vi "autoselect.vi"() -> (1 "60 Goal?":bool, 2 "Offense?":bool)   [LabVIEW 2012, in "Serenity_mk2.lvrbt"]
uses:
  Serenity_mk2.lvrbt
  <vilib>/NXT/Block Support/NXT_ButtonSelector.ctl
  <vilib>/NXT/Dual Mode Library/Display/drawText.vi
  <vilib>/NXT/Dual Mode Library/Sensors/readNXTButton.vi
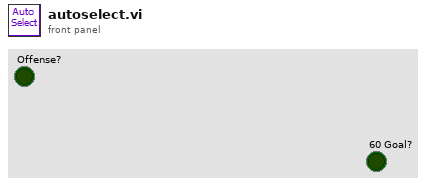
[diagram p1: front panel]
types:
  T1 = typedef "NXT_ButtonSelector.ctl" = u16
  T2 = typedef "LVHSConnector.ctl" = refnum<class "BrickReference.lvclass">
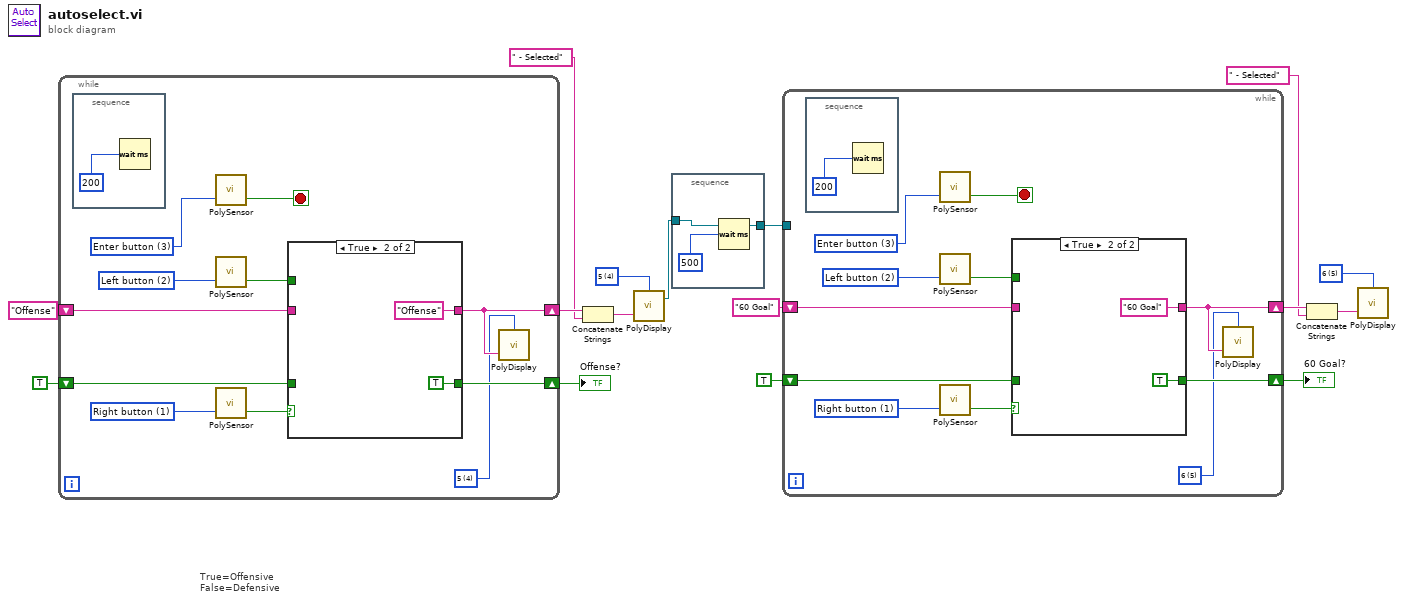
[diagram p0: block diagram]
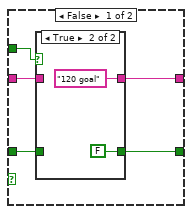
[diagram p2: hidden frame]
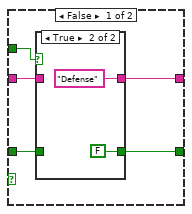
[diagram p4: hidden frame]
diagram:
  w3 = i16 5 items=["1", "2", "3", "4", "5", "6", "7", "8", "9", "10", "11", "12"] ("Line")
  w10 = i16 4 items=["1", "2", "3", "4", "5", "6", "7", "8", "9", "10", "11", "12"] ("Line")
  # "True=Offensive\nFalse=Defensive"
  n1 = while {
    shift-right: [w21] -> w13
    shift-left: "Offense" -> [w25]
    shift-right: [w20] -> w14
    shift-left: TRUE -> [w19]
    stop <- w26 stop-if-true
    w17 = i16 4 items=["1", "2", "3", "4", "5", "6", "7", "8", "9", "10", "11", "12"] ("Line")
    w23 = T1 1 items=["Enter button"=3, "Left button"=2, "Right button"=1, "Up Button"=4, "Down Button"=5] ("Button (Enter button)")
    w24 = T1 2 items=["Enter button"=3, "Left button"=2, "Right button"=1, "Up Button"=4, "Down Button"=5] ("Button (Enter button)")
    w27 = T1 3 items=["Enter button"=3, "Left button"=2, "Right button"=1, "Up Button"=4, "Down Button"=5] ("Button (Enter button)")
    n2 = stacked-sequence {
      frame #0 {
        n3 = Wait (ms)(milliseconds to wait=u32 200 ("Time (1 sec)")) -> ()  [unwired: 1 out]
      }
    }
    n4 = call-poly <vilib>:"PolySensor.vi"("Button (Enter button)"=w27) -> ("Yes/No"=w26:bool)  [unwired: 2 in, 1 out]
    n5 = call-poly <vilib>:"PolySensor.vi"("Button (Enter button)"=w24) -> ("Yes/No"=w18:bool)  [unwired: 2 in, 1 out]
    n6 = call-poly <vilib>:"PolySensor.vi"("Button (Enter button)"=w23) -> ("Yes/No"=w22:bool)  [unwired: 2 in, 1 out]
    n7 = case shown="True" w22 {
      tunnel: w25 -> [w33 _]
      tunnel: [w32 "Offense"] -> w21
      tunnel: [w31 TRUE] -> w20
      tunnel: w19 -> [w30 _]
      tunnel: w18 -> [w29 _]
      frame False {
        n8 = case shown="True" w29 {
          tunnel: w33 -> [w35 _]
          tunnel: [w35 "Defense"] -> w32
          tunnel: [w34 FALSE] -> w31
          tunnel: w30 -> [w34 _]
          frame False {
          }
          frame True {
          }
        }
      }
      frame True {
      }
    }
    n9 = call-poly <vilib>:"PolyDisplay.vi"("Text"=w21, "Line"=w17) -> ()  [unwired: 2 in, 1 out]
  }
  "Offense?" <- w14
  n10 = Concatenate Strings(w13, " - Selected" ("string")) -> (w11:string)
  n11 = call-poly <vilib>:"PolyDisplay.vi"("Text"=w11, "Line"=w10) -> ("NXT/EV3"=w1:T2)  [unwired: 2 in]
  n12 = stacked-sequence {
    tunnel: [w40] -> w2
    tunnel: w1 -> [w40]
    frame #0 {
      n13 = Wait (ms)(milliseconds to wait=u32 500 ("Time (1 sec)")) -> ()  [unwired: 1 out]
    }
  }
  n14 = while {
    shift-right: [w46] -> w6
    shift-left: "60 Goal" -> [w50]
    shift-right: [w45] -> w7
    shift-left: TRUE -> [w44]
    tunnel: w2 -> [_]
    stop <- w51 stop-if-true
    w42 = i16 5 items=["1", "2", "3", "4", "5", "6", "7", "8", "9", "10", "11", "12"] ("Line")
    w48 = T1 1 items=["Enter button"=3, "Left button"=2, "Right button"=1, "Up Button"=4, "Down Button"=5] ("Button (Enter button)")
    w49 = T1 2 items=["Enter button"=3, "Left button"=2, "Right button"=1, "Up Button"=4, "Down Button"=5] ("Button (Enter button)")
    w52 = T1 3 items=["Enter button"=3, "Left button"=2, "Right button"=1, "Up Button"=4, "Down Button"=5] ("Button (Enter button)")
    n15 = stacked-sequence {
      frame #0 {
        n16 = Wait (ms)(milliseconds to wait=u32 200 ("Time (1 sec)")) -> ()  [unwired: 1 out]
      }
    }
    n17 = call-poly <vilib>:"PolySensor.vi"("Button (Enter button)"=w52) -> ("Yes/No"=w51:bool)  [unwired: 2 in, 1 out]
    n18 = call-poly <vilib>:"PolySensor.vi"("Button (Enter button)"=w49) -> ("Yes/No"=w43:bool)  [unwired: 2 in, 1 out]
    n19 = call-poly <vilib>:"PolySensor.vi"("Button (Enter button)"=w48) -> ("Yes/No"=w47:bool)  [unwired: 2 in, 1 out]
    n20 = case shown="True" w47 {
      tunnel: w50 -> [w58 _]
      tunnel: [w57 "60 Goal"] -> w46
      tunnel: [w56 TRUE] -> w45
      tunnel: w44 -> [w55 _]
      tunnel: w43 -> [w54 _]
      frame False {
        n21 = case shown="True" w54 {
          tunnel: w58 -> [w60 _]
          tunnel: [w60 "120 goal"] -> w57
          tunnel: [w59 FALSE] -> w56
          tunnel: w55 -> [w59 _]
          frame False {
          }
          frame True {
          }
        }
      }
      frame True {
      }
    }
    n22 = call-poly <vilib>:"PolyDisplay.vi"("Text"=w46, "Line"=w42) -> ()  [unwired: 2 in, 1 out]
  }
  "60 Goal?" <- w7
  n23 = Concatenate Strings(w6, " - Selected" ("string")) -> (w4:string)
  n24 = call-poly <vilib>:"PolyDisplay.vi"("Text"=w4, "Line"=w3) -> ()  [unwired: 2 in, 1 out]
